vi "FrameCycleTimeSet.vi"(0 "XNET Frame":refnum<k21>, 5 "error in (no error)":errorcluster) -> (14 "MessageFrameCycleTime":i32, 15 "XNET Frame":refnum<k21>, 19 "错误输出":errorcluster)   [LabVIEW 2020]
uses:
  <vilib>/xnet/xnet.llb/XNET Get DBC Mode.ctl
  <vilib>/xnet/xnet.llb/XNET Database Get DBC Attribute (Frame).vi
  <vilib>/Utility/error.llb/Error Cluster From Error Code.vi
  <vilib>/ErrorRing/Error Ring.xnode
  <resource>/objmgr/xnet.rc
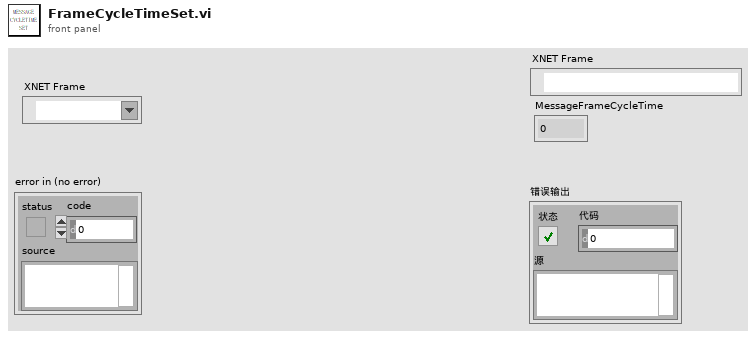
[diagram p1: front panel]
types:
  T1 = typedef "XNET Get DBC Mode.ctl" = u32
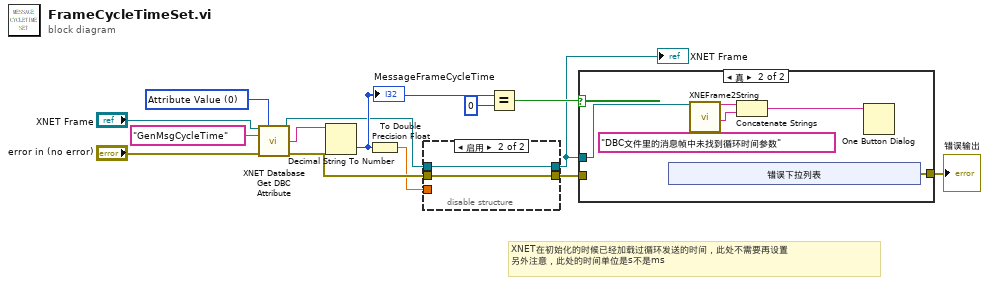
[diagram p0: block diagram]
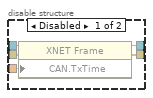
[diagram p2: hidden frame]
diagram:
  w14 = T1 0 items=["Attribute Value", "Enumeration", "Attribute Name List", "Signal Value Table"] ("mode")
  # "XNET在初始化的时候已经加载过循环发送的时间，此处不需要再设置\n另外注意，此处的时间单位是s不是ms"
  n1 = call-poly <vilib>:"XNET Database Get DBC Attribute.vi"("frame in"="XNET Frame", "mode"=w14, "attribute name"="GenMsgCycleTime", "error in (no error)"="error in (no error)") -> ("frame out"=w3:refnum<k21>, "attribute text"=w12:string, "error out"=w11:errorcluster)  [unwired: 8 in, 1 out]
  n2 = Decimal String To Number(string=w12) -> (number=w8:i32)  [unwired: 2 in, 1 out]
  "MessageFrameCycleTime" <- w8
  n3 = To Double Precision Float(number=w8) -> (double precision float=w9:dbl)
  n4 = disable-structure shown="启用" {
    disable-tunnel: w11 -> [w19 w20]
    disable-tunnel: w9 -> [w18 _]
    disable-tunnel: [w17 w20] -> w5
    disable-tunnel: w3 -> [w16 w21]
    disable-tunnel: [w15 w21] -> w1
    frame Disabled {
      n5 = property class="XNET Frame"(reference=w16, error in=w19, "CAN.TxTime"=w18) -> (reference out=w15:refnum<k21>, error out=w17:errorcluster)
    }
    frame Enabled {
    }
  }
  "XNET Frame" <- w1
  n6 = Equal?(x=w8, y=0) -> (x = y?=w6:bool)
  n7 = case shown="真" w6 {
    tunnel: w5 -> [w22 _]
    tunnel: [w22 w27] -> w2
    tunnel: w1 -> [_ w26]
    frame False {
    }
    frame True {
      n8 = xnode "错误下拉列表"() -> ("错误输出"=w27:errorcluster)
      n9 = call "XNEFrame2String.vi"("XNET Frame"=w26) -> ("X-netString"=w25:string)  [unwired: 18 in]
      n10 = Concatenate Strings(w25, "DBC文件里的消息帧中未找到循环时间参数" ("消息")) -> (w23:string)
      n11 = One Button Dialog(message=w23) -> ()  [unwired: 1 in, 1 out]
    }
  }
  "错误输出" <- w2
